vi "Test To Report Entry.vi"(8 "error in (no error)":errorcluster, 9 "Asserts (aka. Test Cases)":T4[](array[typedef]), 10 "Node (aka. Test Suite)":T5) -> (0 "error out":errorcluster, 1 "testcases":T1[](array[typedef]), 2 "testsuite":T2)   [LabVIEW 2009, in "Caraya.lvlib" / "Test Report.JUnit.lvclass"]
uses:
  Test Report.JUnit.lvclass
  Test Event Storage/Test Node.ctl
  Basic Test Manager/Test Registration Data.ctl
  Basic Test Manager/Assert Event Data.ctl
  testsuite -- cluster.ctl
  property -- cluster.ctl
  testcase -- cluster.ctl
  Basic Test Manager/Basic Test Manager.lvclass
  Test Event Storage/Test Event Storage.lvclass
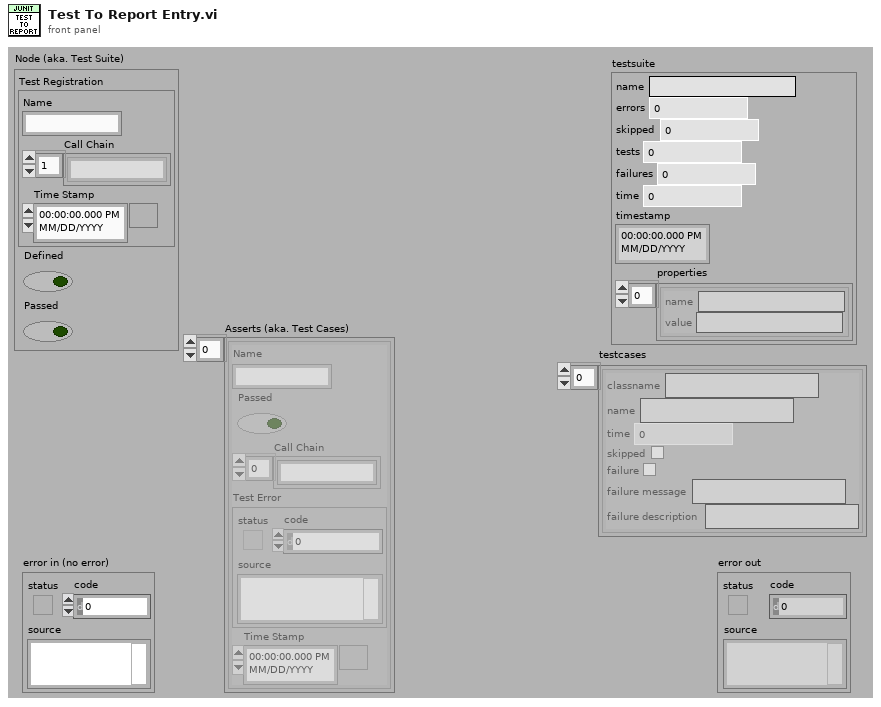
[diagram p1: front panel]
types:
  T1 = typedef "Caraya.lvlib/Test Report.JUnit.lvclass/testcase -- cluster.ctl" = cluster{"classname":string, "name":string, "time":dbl, "skipped":bool, "failure":bool, "failure message":string, "failure description":string}
  T2 = typedef "Caraya.lvlib/Test Report.JUnit.lvclass/testsuite -- cluster.ctl" = cluster{"name":string, "errors":u32, "skipped":u32, "tests":u32, "failures":u32, "time":dbl, "timestamp":timestamp, "properties":T3[]}
  T3 = typedef "property -- cluster.ctl" = cluster{"name":string, "value":string}
  T4 = typedef "Caraya.lvlib/Basic Test Manager.lvclass/Assert Event Data.ctl" = cluster{"Name":string, "Passed":bool, "Call Chain":string[], "Test Error":errorcluster, "Time Stamp":timestamp}
  T5 = typedef "Caraya.lvlib/Test Event Storage.lvclass/Test Node.ctl" = cluster{"Test Registration":T6, "Defined":bool, "Passed":bool}
  T6 = typedef "Caraya.lvlib/Basic Test Manager.lvclass/Test Registration Data.ctl" = cluster{"Name":string, "Call Chain":string[], "Time Stamp":timestamp}
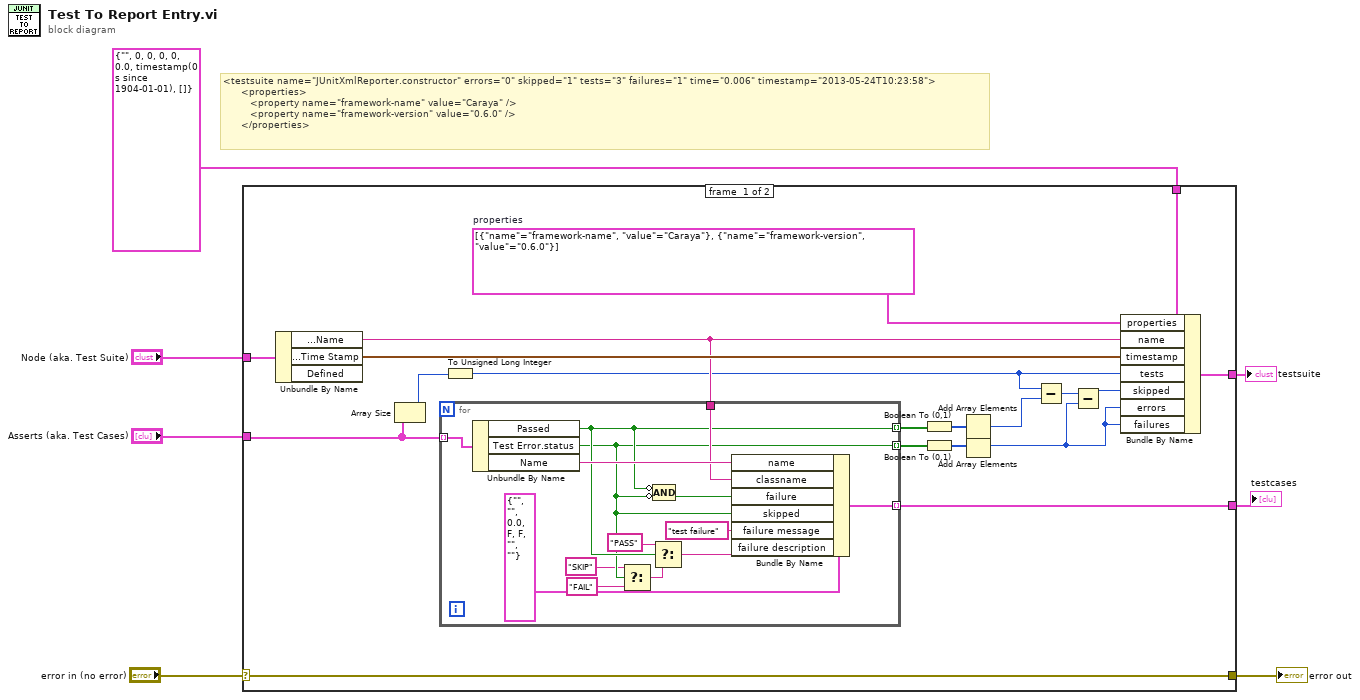
[diagram p0: block diagram]
diagram:
  # "<testsuite name=\"JUnitXmlReporter.constructor\" errors=\"0\" skipped=\"1\" tests=\"3\" failures=\"1\" time=\"0.006\" timestamp=\"2013-05-24T10:23:58\">\n      <properties>\n         <property name=\"framework-name\" value=\"Caraya\" />\n         <property name=\"framework-version\" value=\"0.6.0\" />\n      </properties>"
  n1 = case shown="No Error" "error in (no error)" {
    selector: "error in (no error)" -> [w25 w41]
    tunnel: [w25 w41] -> w6
    tunnel: "Node (aka. Test Suite)" -> [w26 _]
    tunnel: T2 {"name"="", "errors"=0, "skipped"=0, "tests"=0, "failures"=0, "time"=0.0, "timestamp"=timestamp(0 s since 1904-01-01), "properties"=[]} ("testsuite") -> [w24 _]
    tunnel: "Asserts (aka. Test Cases)" -> [w22 _]
    tunnel: [w16 _] -> w2
    tunnel: [w13 _] -> w1
    frame #0 {
      w15 = T3[] [{"name"="framework-name", "value"="Caraya"}, {"name"="framework-version", "value"="0.6.0"}]  # properties
      n2 = Unbundle By Name(w26) -> ("Test Registration.Name"=w14:string, "Test Registration.Time Stamp"=w23:timestamp)  [unwired: 1 out]
      n3 = Array Size(array=w22) -> (size(s)=w20:i32)
      n4 = for {
        tunnel: w22 -> [w40] mode=indexing
        tunnel: [w33] -> w21 mode=indexing
        tunnel: [w30] -> w9 mode=indexing
        tunnel: w14 -> [w37]
        tunnel: [w34] -> w13 mode=indexing
        n5 = Unbundle By Name(w40) -> ("Passed"=w33:bool, "Test Error.status"=w30:bool, "Name"=w38:string)
        n6 = Select(t="SKIP" ("failure message"), s=w30, f="FAIL" ("failure message")) -> (s? t:f=w29:string)
        n7 = Compound Arithmetic op=AND(invert w33, invert w30) -> (w36:bool)
        n8 = Select(t="PASS" ("failure message"), s=w33, f=w29) -> (s? t:f=w32:string)
        n9 = Bundle By Name(cluster=T1 {"classname"="", "name"="", "time"=0.0, "skipped"=FALSE, "failure"=FALSE, "failure message"="", "failure description"=""} ("testcase"), "name"=w38, "classname"=w37, "failure"=w36, "skipped"=w30, "failure message"="test failure", "failure description"=w32) -> (w34:T1)
      }
      n10 = To Unsigned Long Integer(number=w20) -> (unsigned 32bit integer=w12:u32)
      n11 = Boolean To (0,1)(Boolean=w21) -> (0, 1=w19:i16[])
      n12 = Boolean To (0,1)(Boolean=w9) -> (0, 1=w10:i16[])
      n13 = Add Array Elements(numeric array=w19) -> (sum=w11:i16)
      n14 = Add Array Elements(numeric array=w10) -> (sum=w8:i16)
      n15 = Subtract(x=w12, y=w11) -> (x-y=w18:u32)
      n16 = Subtract(x=w18, y=w8) -> (x-y=w17:u32)
      n17 = Bundle By Name(cluster=w24, "properties"=w15, "name"=w14, "timestamp"=w23, "tests"=w12, "skipped"=w17, "errors"=w8, "failures"=w8) -> (w16:T2)
    }
    frame #1 {
    }
  }
  "error out" <- w6
  "testsuite" <- w2
  "testcases" <- w1
